vi "assembly_amp_0dB_result.vi"(2 "meas_koef_0_0":dbl[][](array[numeric]), 3 "boc_data_koef_0_0":sgl[][](array[numeric]), 5 "meas_koef_0_3":dbl[][](array[numeric]), 6 "meas_koef_-1_0":dbl[][](array[numeric]), 7 "boc_data_koef_0_3":sgl[][](array[numeric]), 8 "error in (no error)":errorcluster, 9 "boc_data_koef_-1_0":sgl[][](array[numeric]), 10 "meas_koef_-1_3":dbl[][](array[numeric]), 11 "boc_data_koef_-1_3":sgl[][](array[numeric])) -> (0 "error out":errorcluster)   [LabVIEW 2017]
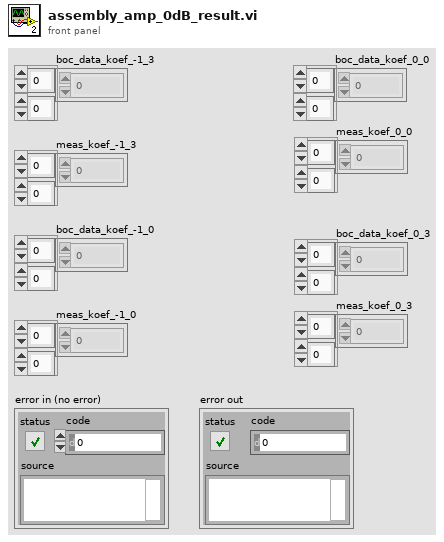
[diagram p1: front panel]
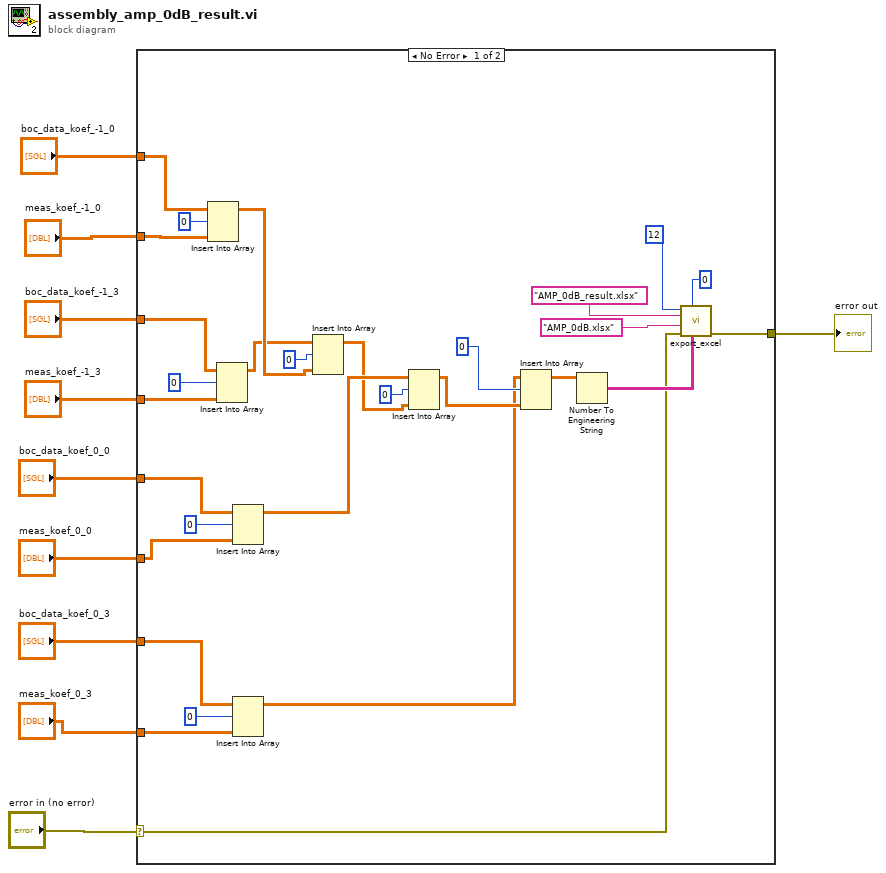
[diagram p0: block diagram]
diagram:
  n1 = case shown="No Error" "error in (no error)" {
    selector: "error in (no error)" -> [w27 w40]
    tunnel: [w36 w40] -> w10
    tunnel: "meas_koef_-1_3" -> [w34 _]
    tunnel: "boc_data_koef_-1_3" -> [w33 _]
    tunnel: "meas_koef_-1_0" -> [w30 _]
    tunnel: "boc_data_koef_-1_0" -> [w29 _]
    tunnel: "boc_data_koef_0_0" -> [w24 _]
    tunnel: "meas_koef_0_0" -> [w23 _]
    tunnel: "boc_data_koef_0_3" -> [w16 _]
    tunnel: "meas_koef_0_3" -> [w15 _]
    frame No Error {
      n2 = Insert Into Array(array=w29, index (row)=0, new element=w30) -> (w21:sgl[][])  [unwired: 1 in]
      n3 = Insert Into Array(array=w33, index (row)=0, new element=w34) -> (w20:sgl[][])  [unwired: 1 in]
      n4 = Insert Into Array(array=w24, index (row)=0, new element=w23) -> (w19:sgl[][])  [unwired: 1 in]
      n5 = Insert Into Array(array=w16, index (row)=0, new element=w15) -> (w11:sgl[][])  [unwired: 1 in]
      n6 = Insert Into Array(array=w20, index (row)=0 ("disabled index (col)"), new element=w21) -> (w18:sgl[][])  [unwired: 1 in]
      n7 = Insert Into Array(array=w19, index (row)=0 ("disabled index (col)"), new element=w18) -> (w12:sgl[][])  [unwired: 1 in]
      n8 = Insert Into Array(array=w11, index (row)=0 ("disabled index (col)"), new element=w12) -> (w13:sgl[][])  [unwired: 1 in]
      n9 = Number To Engineering String(4:w13) -> (0:w35:string[][])  [unwired: 3 in]
      n10 = call "export_excel.vi"("table"=w35, "position (excel).row"=0, "error in (no error)"=w27, "template_filename"="AMP_0dB.xlsx", "result_filename"="AMP_0dB_result.xlsx", "position (excel).column"=12) -> ("error out"=w36:errorcluster)  [unwired: 5 in]
    }
    frame Error {
    }
  }
  "error out" <- w10
